vi "Motion Track.vi"(0 "vel":dbl, 5 "Kv":dbl=0.09 format="%#_13g", 7 "acc":dbl, 9 "Ka":dbl=0.02 format="%#_13g", 11 "error":dbl, 12 "PID Settings":T1) -> (4 "Power":dbl)   [LabVIEW 2015]
uses:
  Support/LightningPID Settings.ctl
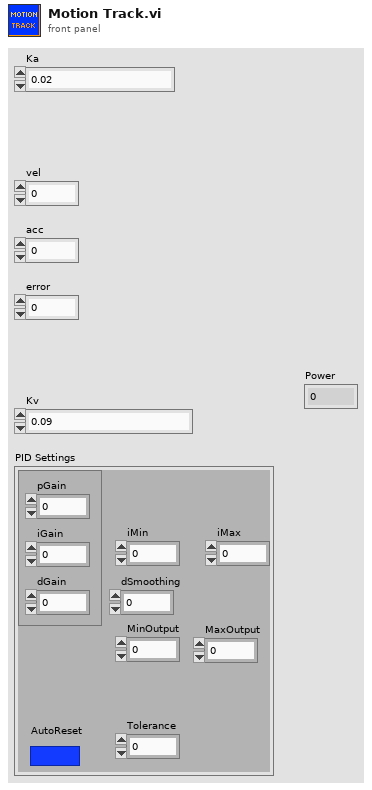
[diagram p1: front panel]
types:
  T1 = typedef "LightningPID Settings.ctl" = cluster{"iMax":dbl, "iMin":dbl, "iGain":dbl, "pGain":dbl, "dGain":dbl, "MaxOutput":dbl, "MinOutput":dbl, "AutoReset":bool, "Tolerance":dbl, "dSmoothing":dbl}
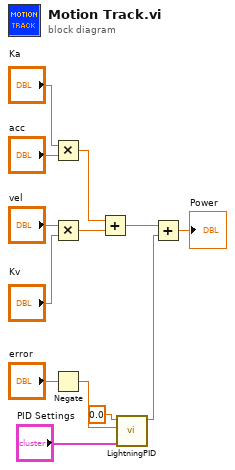
[diagram p0: block diagram]
diagram:
  n1 = Multiply(x="Ka", y="acc") -> (x*y=w7:dbl)
  n2 = Multiply(x="vel", y="Kv") -> (x*y=w8:dbl)
  n3 = Negate(x="error") -> (-x=w2:dbl)
  n4 = Add(x=w7, y=w8) -> (x+y=w9:dbl)
  n5 = call "LightningPID.vi"("PID Settings"="PID Settings", "Position"=w2, "Set Point"=0.0) -> ("Output"=w13:dbl)  [unwired: 8 in]
  n6 = Add(x=w9, y=w13) -> (x+y=→"Power":dbl)
